vi "ConfigureFreeRunning.vi"(0 "object in":refnum<class "Hamamatsu.lvclass">, 5 "error in (no error)":errorcluster) -> (14 "object out":refnum<class "Hamamatsu.lvclass">, 19 "error out":errorcluster)   [LabVIEW 2021, in "Hamamatsu.lvclass"]
uses:
  Hamamatsu.lvclass
  Hamamatsu.lvclass/Hamamatsu.ctl
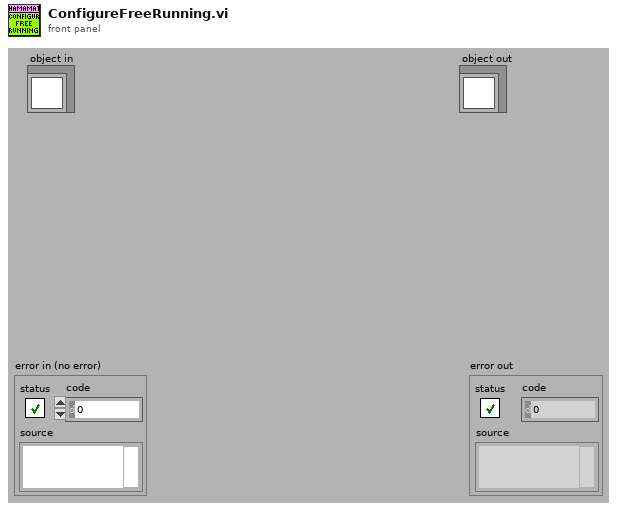
[diagram p1: front panel]
types:
  T1 = typedef "IMAQ Image.ctl" = refnum<image>
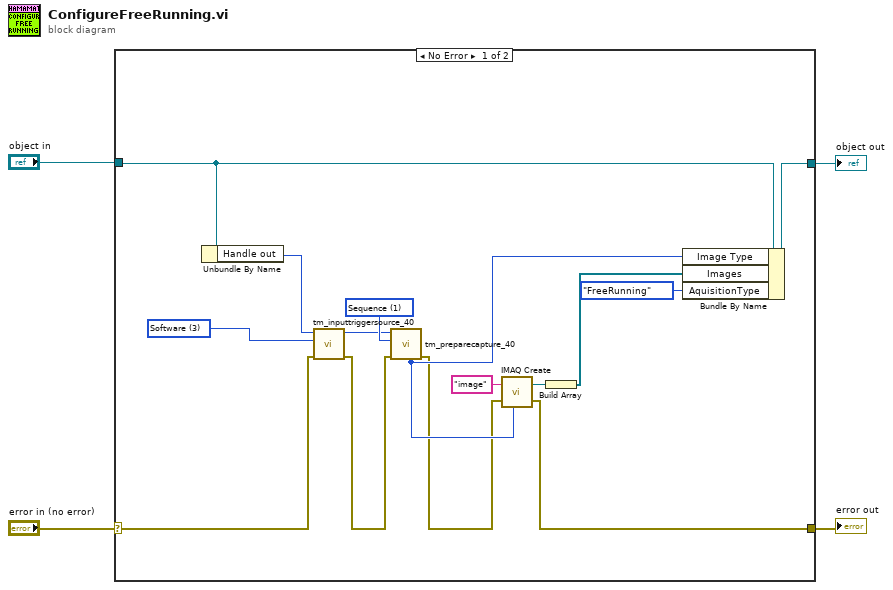
[diagram p0: block diagram]
diagram:
  n1 = case shown="No Error" "error in (no error)" {
    selector: "error in (no error)" -> [w10 w21]
    tunnel: [w14 w21] -> w3
    tunnel: [w18 w20] -> w1
    tunnel: "object in" -> [w19 w20]
    frame No Error {
      w8 = 3 items=["Internal"=1, "External"=2, "Software"=3, "Master Pulse"=4] ("Source")
      w17 = 1 items=["Snap", "Sequence"] ("Capture mode")
      n2 = Unbundle By Name(w19) -> ("Handle out"=w12:u32)
      n3 = call <userlib>:"tm_inputtriggersource_40.vi"("error in (no error)"=w10, "Source"=w8, "Handle in"=w12) -> ("error out"=w9:errorcluster, "Handle out"=w11:u32)  [unwired: 7 in]
      n4 = call <userlib>:"tm_preparecapture_40.vi"("error in (no error)"=w9, "Capture mode"=w17, "Handle in"=w11) -> ("error out"=w13:errorcluster, "Image type"=w15:u32)  [unwired: 5 in, 2 out]
      n5 = call "IMAQ Create"("Image Name"="image", "Image Type"=w15, "error in (no error)"=w13) -> ("New Image"=w7:T1, "error out"=w14:errorcluster)  [unwired: 2 in]
      n6 = Build Array(w7) -> (w6:T1[])
      n7 = Bundle By Name(cluster=w19, "Image Type"=w15, "Images"=w6, "AquisitionType"=enum16{"HWSynced", "FreeRunning"}."FreeRunning") -> (w18:refnum<class "Hamamatsu.lvclass">)
    }
    frame Error {
    }
  }
  "error out" <- w3
  "object out" <- w1
